vi "DE_SHAPE_REPORT_A_MATCHES(SubVI).vi"(1 "Shape Report":T2(array[cluster])) -> (0 "Matches":T1(array[cluster]) {"Bounding Box"."y" format="%.2f"; "Bounding Box"."x" format="%.2f"; "Position"."y" format="%.2f"; "Position"."x" format="%.2f"; "Score" format="%.2f"; "Scale" format="%.2f"; "Angle" format="%.2f"})   [LabVIEW 2011]
doc: "cambia DE SHAPE REPORT A MATCHES, para poder en encajar los datos de shape de global rectangle a bunding box y de centroid a position; otros cambias de object Size a Scale, angle ninguno (360 defecto), Score a Score."
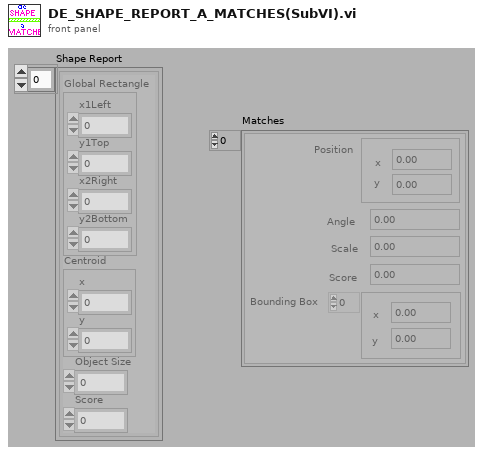
[diagram p1: front panel]
types:
  T1 = cluster{"Position":cluster{"x":sgl, "y":sgl}, "Angle":sgl, "Scale":sgl, "Score":sgl, "Bounding Box":cluster{"x":sgl, "y":sgl}[]}[]
  T2 = cluster{"Global Rectangle":cluster{"x1Left":i32, "y1Top":i32, "x2Right":i32, "y2Bottom":i32}, "Centroid":cluster{"x":sgl, "y":sgl}, "Object Size":u32, "Score":dbl}[]
  T3 = cluster{"x1Left":i32, "y1Top":i32, "x2Right":i32, "y2Bottom":i32}
  T4 = cluster{"Position":cluster{"x":sgl, "y":sgl}, "Angle":sgl, "Object Size":u32, "Score":dbl, cluster{sgl, sgl}[]}
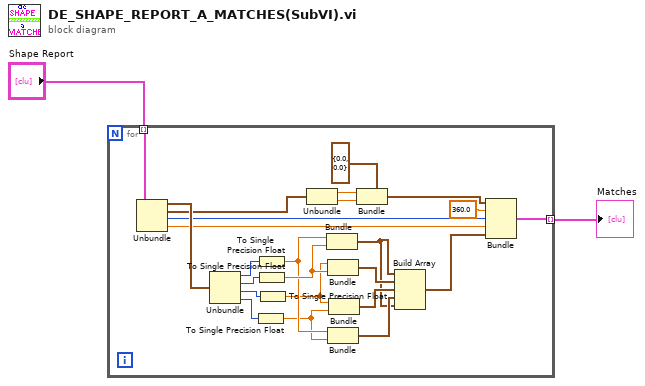
[diagram p0: block diagram]
diagram:
  n1 = for {
    tunnel: "Shape Report" -> [w26] mode=indexing
    tunnel: [w25] -> w1 mode=indexing
    n2 = Unbundle(w26) -> ("Global Rectangle"=w24:T3, "Centroid"=w23:cluster{"x":sgl, "y":sgl}, "Object Size"=w22:u32, "Score"=w21:dbl)
    n3 = Unbundle(w24) -> ("x1Left"=w13:i32, "y1Top"=w14:i32, "x2Right"=w15:i32, "y2Bottom"=w12:i32)
    n4 = To Single Precision Float(number=w12) -> (single precision float=w9:sgl)
    n5 = To Single Precision Float(number=w13) -> (single precision float=w10:sgl)
    n6 = To Single Precision Float(number=w14) -> (single precision float=w11:sgl)
    n7 = To Single Precision Float(number=w15) -> (single precision float=w8:sgl)
    n8 = Unbundle(w23) -> ("x"=w18:sgl, "y"=w17:sgl)
    n9 = Bundle(w10, w11) -> (w3:cluster{sgl, sgl})  [unwired: 1 out]
    n10 = Bundle(w8, w11) -> (w7:cluster{sgl, sgl})  [unwired: 1 out]
    n11 = Bundle(w10, w9) -> (w5:cluster{sgl, sgl})  [unwired: 1 out]
    n12 = Bundle(w8, w9) -> (w6:cluster{sgl, sgl})  [unwired: 1 out]
    n13 = Bundle(cluster=cluster{"x":sgl, "y":sgl} {"x"=0.0, "y"=0.0} ("Position"), "x"=w18, "y"=w17) -> (w16:cluster{"x":sgl, "y":sgl})
    n14 = Build Array(w3, w7, w6, w5, w3) -> (w4:cluster{sgl, sgl}[])
    n15 = Bundle("Position"=w16, "Angle"=sgl 360.0, "Object Size"=w22, "Score"=w21, w4) -> (w25:T4)  [unwired: 1 out]
  }
  "Matches" <- w1
